vi "mkConfigureBufferList.vi"(10 "Camera in":T1={"Gain [1-4]"=10.0, "Offset"=1, "Mode"=75, "ROIs"=[], "ROI Size"={"X"=0, "Y"=0}, "Number of buffers"=40, "Use hardware multiple-ROI?"=TRUE, "GenericCameraConfig"={"Framerate (Hz)"=60, "Exposure time (us)"=5000, "Image size"={"Width"=1280, "Height"=1024}, "Number of buffers"=30}}, 11 "IMAQ Session":refnum<k11>) -> (3 "IMAQ Session (out)":refnum<k11>)   [LabVIEW 2011]
uses:
  CameraConfig.ctl
  Main/Camera/GenericCameraConfigType.ctl
panel:
  # "us"
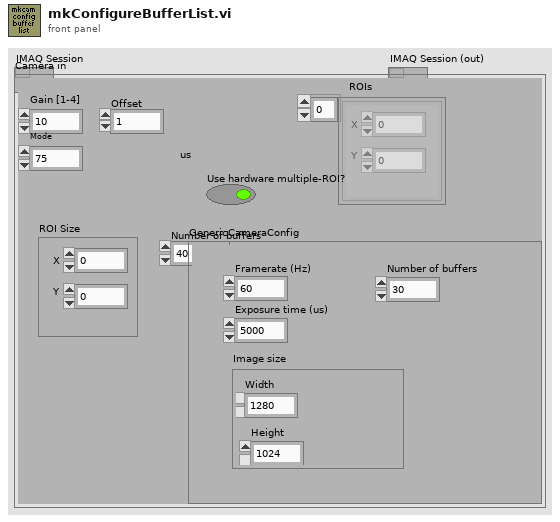
[diagram p1: front panel]
types:
  T1 = typedef "CameraConfig.ctl" = cluster{"Gain [1-4]":sgl, "Offset":i16, "Mode":i16, "ROIs":cluster{"X":i32, "Y":i32}[], "ROI Size":cluster{"X":i32, "Y":i32}, "Number of buffers":i32, "Use hardware multiple-ROI?":bool, "GenericCameraConfig":T2}
  T2 = typedef "GenericCameraConfigType.ctl" = cluster{"Framerate (Hz)":i32, "Exposure time (us)":i32, "Image size":cluster{"Width":i32, "Height":i32}, "Number of buffers":i32}
  T3 = typedef "Image Type" = u32
  T4 = typedef "IMAQ Image.ctl" = refnum<image>
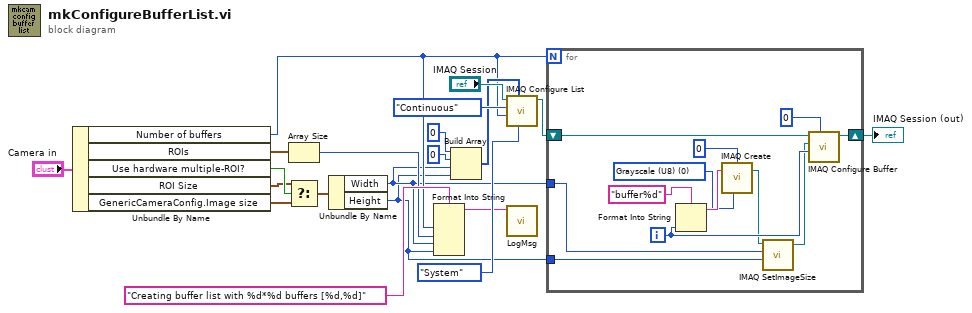
[diagram p0: block diagram]
diagram:
  n1 = Unbundle By Name("Camera in") -> ("Number of buffers"=w9:i32, "ROIs"=w8:cluster{"X":i32, "Y":i32}[], "Use hardware multiple-ROI?"=w6:bool, "ROI Size"=w5:cluster{"X":i32, "Y":i32}, "GenericCameraConfig.Image size"=w4:cluster{"Width":i32, "Height":i32})
  n2 = Array Size(array=w8) -> (size(s)=w7:i32)
  n3 = Select(t=w5, s=w6, f=w4) -> (s? t:f=w3:cluster{"Width":i32, "Height":i32})
  n4 = Unbundle By Name(w3) -> ("Width"=w2:i32, "Height"=w1:i32)
  n5 = Format Into String(format string="Creating buffer list with %d*%d buffers [%d,%d]" ("msg"), w9, w7, w2, w1) -> (resulting string=w10:string)  [unwired: 2 in, 1 out]
  n6 = Build Array(0 ("element"), 0 ("element"), w2, w1) -> (w15:i32[])
  n7 = call <vilib>:"IMAQ Configure List.vi"("Memory Location"=enum16{"System", "Onboard"}."System", "Region of interest"=w15, "Number of buffers"=w9, "Continuous?"=enum16{"One-Shot", "Continuous"}."Continuous", "IMAQ Session In"="IMAQ Session") -> ("IMAQ Session Out"=w13:refnum<k11>)  [unwired: 5 in, 1 out]
  n8 = call "LogMsg.vi"("msg"=w10) -> ()  [unwired: 11 in]
  n9 = for {
    N: w9 -> [_]
    shift-right: [w25] -> w12
    shift-left: w13 -> [w32]
    tunnel: w2 -> [w22]
    tunnel: w1 -> [w21]
    i -> [w27]
    w29 = T3 0 items=["Grayscale (U8)", "Grayscale (I16)", "Grayscale (SGL)", "Complex (CSG)", "RGB (U32)", "HSL (U32)", "RGB (U64)", "Grayscale (U16)"] ("Image Type")
    n10 = Format Into String(format string="buffer%d" ("Image Name"), w27) -> (resulting string=w30:string)  [unwired: 2 in, 1 out]
    n11 = call "IMAQ Create"("Border Size"=0, "Image Name"=w30, "Image Type"=w29) -> ("New Image"=w24:T4)  [unwired: 2 in, 1 out]
    n12 = call "IMAQ SetImageSize"("Y Resolution"=w21, "X Resolution"=w22, "Image"=w24) -> ("Image Out"=w23:T4)  [unwired: 2 in, 1 out]
    n13 = call <vilib>:"IMAQ Configure Buffer.vi"("Skip Count"=u32 0, "Buffer Number"=w27, "Image In"=w23, "IMAQ Session In"=w32) -> ("IMAQ Session Out"=w25:refnum<k11>)  [unwired: 6 in, 1 out]
  }
  "IMAQ Session (out)" <- w12
